vi "StressDist_plot.vi"(7 "StressDist_types":T8, 8 "Error In":errorcluster, 11 "main_FGV_data":T1={"pipe_properties"={"out_radius"=0.0, "in_radius"=0.0, "out_diameter"=0.0, "in_diameter"=0.0, "thickness"=0.0, "inertia"=0.0, "area"=0.0}, "DirPath"=path "L:/Documentos/00 SERVIÇOS/Tensão residual/Olapa 10-2017/Dados/Primeira Seção/Furos", "DirReport"=path "L:/Documentos/00 SERVIÇOS/Tensão residual/Olapa 10-2017/RelatóriosOlapa/Teste", "Points"=[], "ovalization_data"={"AngOval"=[0.0, 60.0, 120.0, 22.5, 45.0, 67.5, 90.0, 112.5, 135.0, 157.5, 180.0], "OvalDiam"=[324.25, 324.6, 324.55, 324.25, 324.55, 324.65, 324.6, 324.65, 324.55, 324.5, 324.4], "Plots"={"Ref"={"X"=[], "Y"=[]}, "Elipse"={"X"=[], "Y"=[]}, "Points"={"X"=[], "Y"=[]}}, "Ampliation"=100.0, "Results"={"MD"=0.0, "mD"=0.0, "Dmed"=0.0, "Oval"=0.0, "ang"=0.0, "X0"=0.0, "Y0"=0.0}}, "StressDist_data"={"Long"={"Plot"=[], "Fit"=[], "ColorMap"=[], "Data"=[], "peirce_data"={"Plot"=[], "Index removidos"=[]}}, "Circ"={"Plot"=[], "Fit"=[], "ColorMap"=[], "Data"=[], "peirce_data"={"Plot"=[], "Index removidos"=[]}}, "Shear"={"Plot"=[], "Fit"=[], "ColorMap"=[], "Data"=[], "peirce_data"={"Plot"=[], "Index removidos"=[]}}}}) -> (0 "Error Out":errorcluster, 3 "main_FGV_data-out":T1={"pipe_properties"={"out_radius"=0.0, "in_radius"=0.0, "out_diameter"=0.0, "in_diameter"=0.0, "thickness"=0.0, "inertia"=0.0, "area"=0.0}, "DirPath"=path "L:/Documentos/00 SERVIÇOS/Tensão residual/Olapa 10-2017/Dados/Primeira Seção/Furos", "DirReport"=path "L:/Documentos/00 SERVIÇOS/Tensão residual/Olapa 10-2017/RelatóriosOlapa/Teste", "Points"=[], "ovalization_data"={"AngOval"=[0.0, 60.0, 120.0, 22.5, 45.0, 67.5, 90.0, 112.5, 135.0, 157.5, 180.0], "OvalDiam"=[324.25, 324.6, 324.55, 324.25, 324.55, 324.65, 324.6, 324.65, 324.55, 324.5, 324.4], "Plots"={"Ref"={"X"=[], "Y"=[]}, "Elipse"={"X"=[], "Y"=[]}, "Points"={"X"=[], "Y"=[]}}, "Ampliation"=100.0, "Results"={"MD"=0.0, "mD"=0.0, "Dmed"=0.0, "Oval"=0.0, "ang"=0.0, "X0"=0.0, "Y0"=0.0}}, "StressDist_data"={"Long"={"Plot"=[], "Fit"=[], "ColorMap"=[], "Data"=[], "peirce_data"={"Plot"=[], "Index removidos"=[]}}, "Circ"={"Plot"=[], "Fit"=[], "ColorMap"=[], "Data"=[], "peirce_data"={"Plot"=[], "Index removidos"=[]}}, "Shear"={"Plot"=[], "Fit"=[], "ColorMap"=[], "Data"=[], "peirce_data"={"Plot"=[], "Index removidos"=[]}}}})   [LabVIEW 2016]
uses:
  StressDist_types.ctl
  MainFGV/main_FGV_data.ctl
  MainFGV/pipe_properties.ctl
  StressCalculations/point_data.ctl
  Ovalization/ovalization_data.ctl
  StressDist_data.ctl
  StressDist_single_data.ctl
  Peirce/peirce_data.ctl
  <vilib>/Analysis/1siggen.llb/Ramp Pattern by Samples.vi
  <vilib>/Analysis/NI_AALBase.lvlib
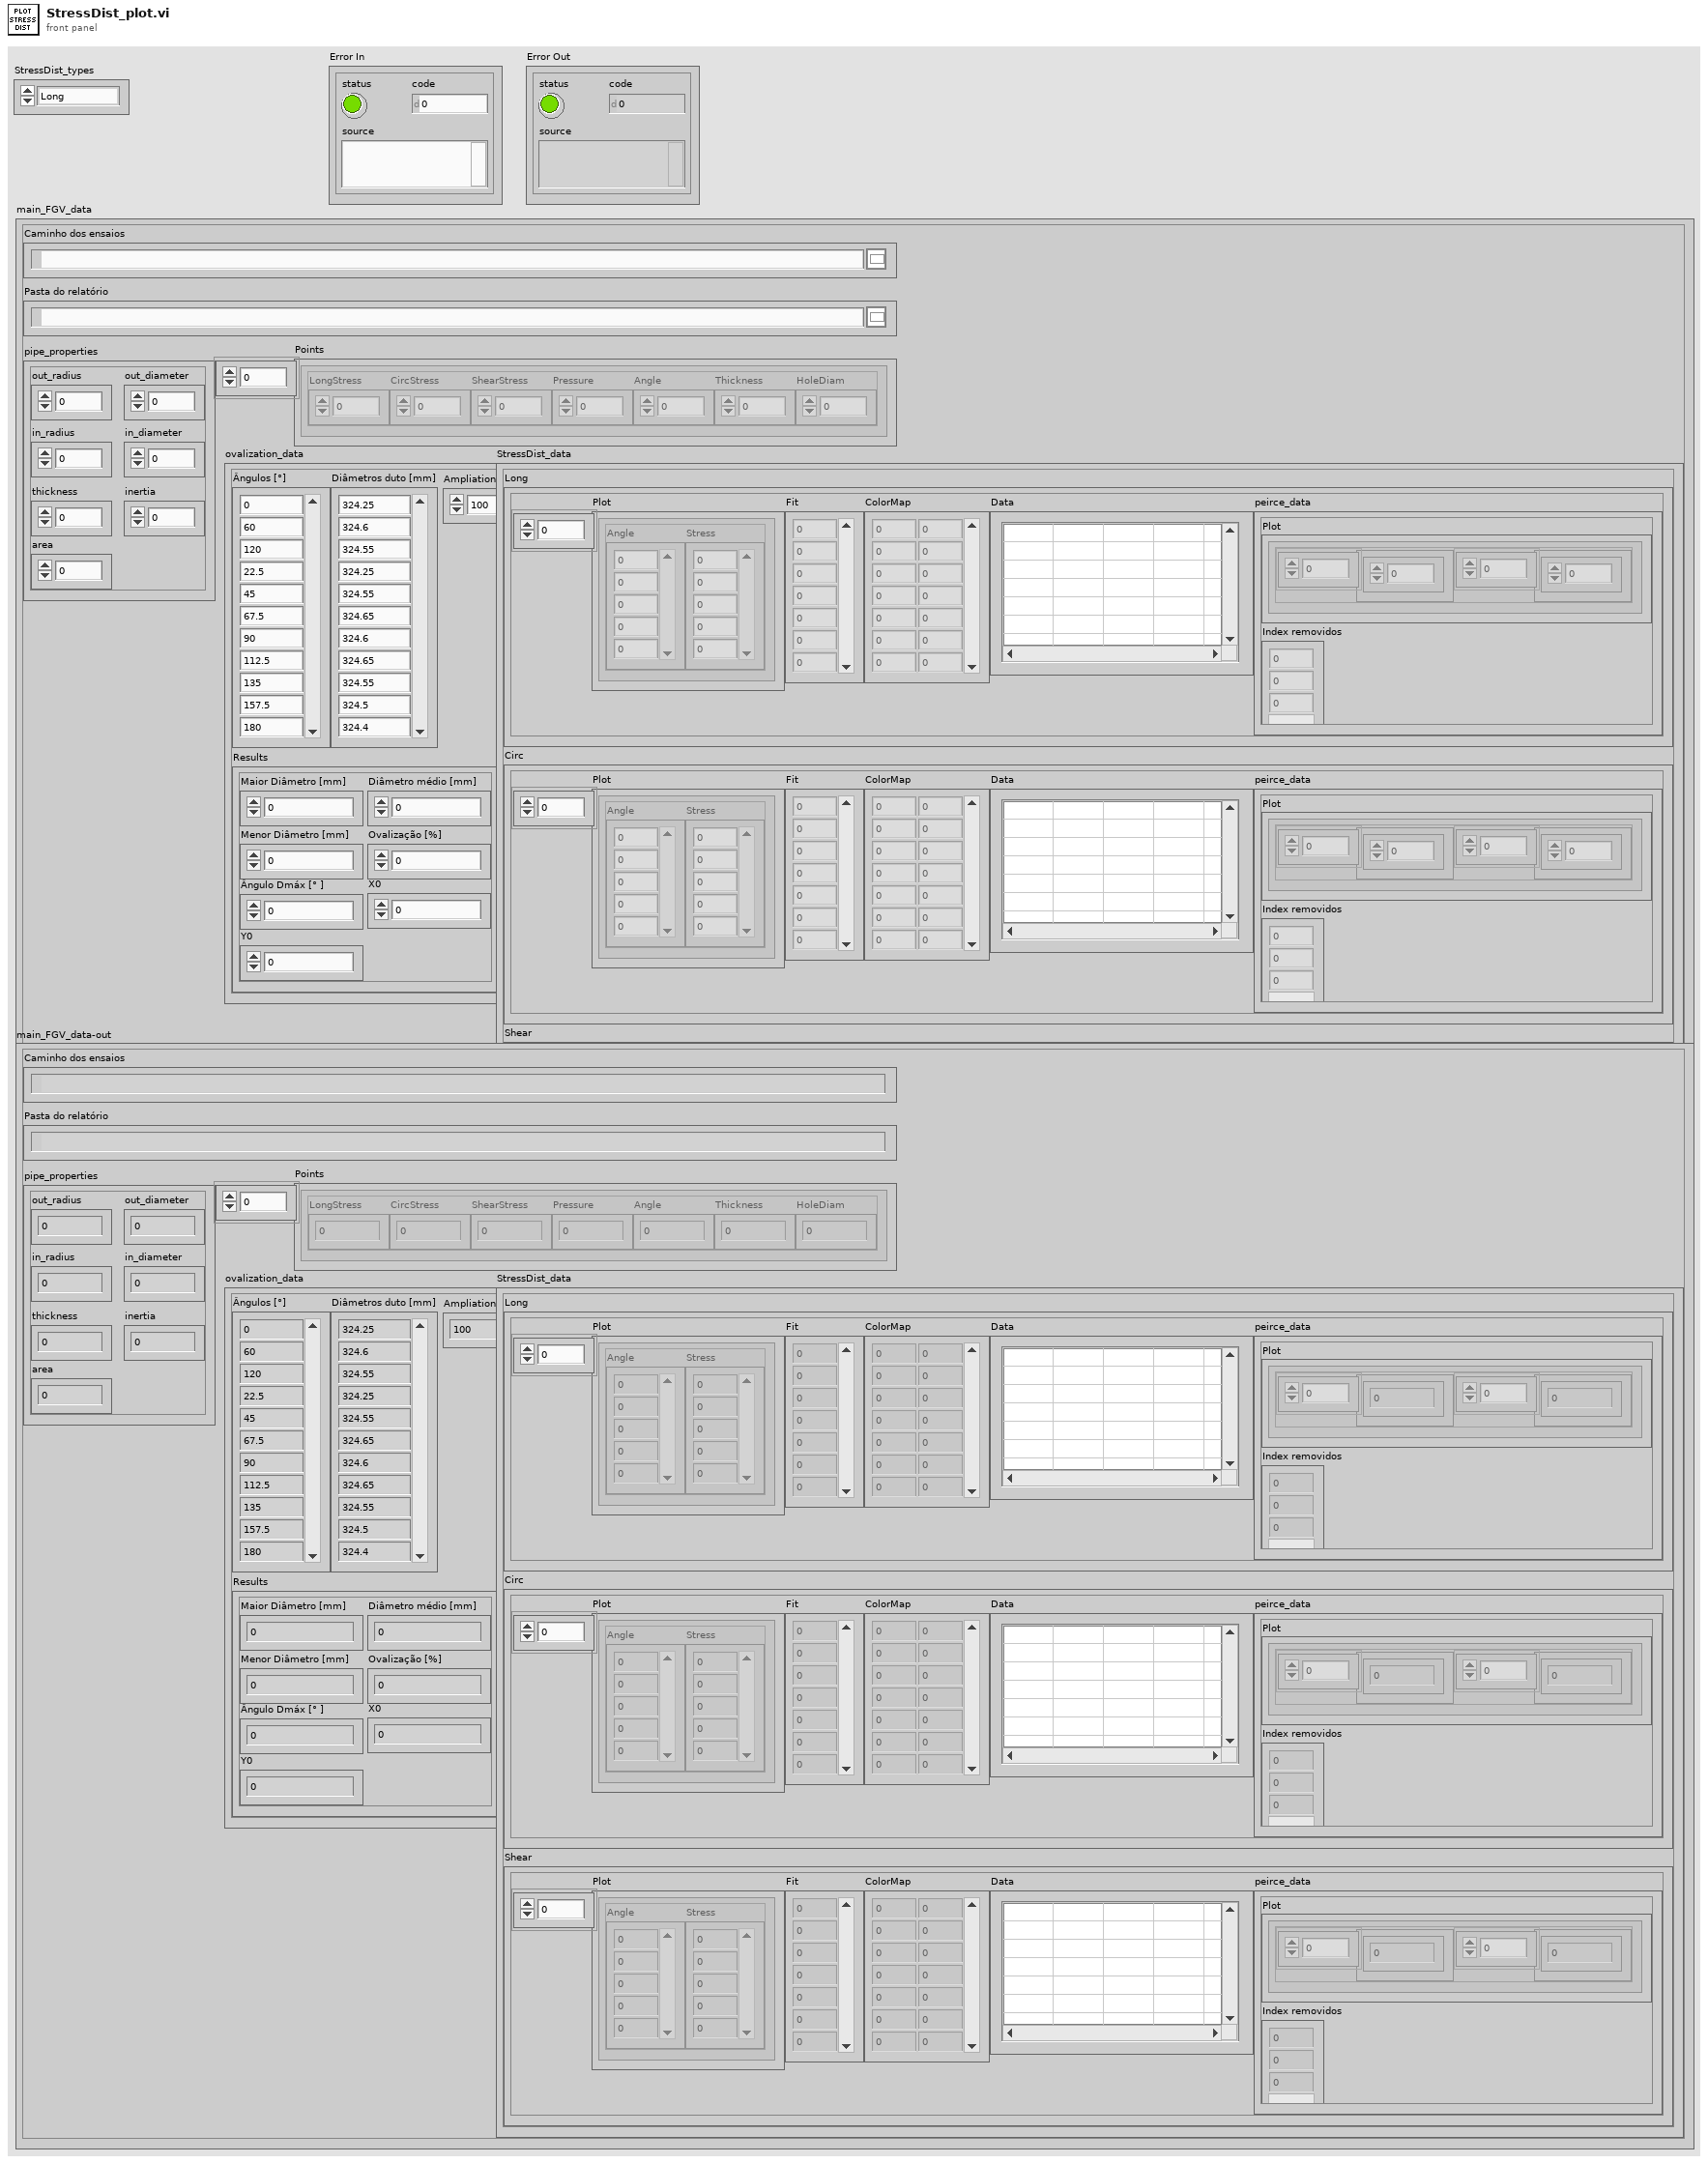
[diagram p1: front panel]
types:
  T1 = typedef "main_FGV_data.ctl" = cluster{"pipe_properties":T2, "DirPath":path, "DirReport":path, "Points":T3[], "ovalization_data":T4, "StressDist_data":T5}
  T2 = typedef "pipe_properties.ctl" = cluster{"out_radius":dbl, "in_radius":dbl, "out_diameter":dbl, "in_diameter":dbl, "thickness":dbl, "inertia":dbl, "area":dbl}
  T3 = typedef "point_data.ctl" = cluster{"LongStress":dbl, "CircStress":dbl, "ShearStress":dbl, "Pressure":dbl, "Angle":dbl, "Thickness":dbl, "HoleDiam":dbl}
  T4 = typedef "ovalization_data.ctl" = cluster{"AngOval":dbl[], "OvalDiam":dbl[], "Plots":cluster{"Ref":cluster{"X":dbl[], "Y":dbl[]}, "Elipse":cluster{"X":dbl[], "Y":dbl[]}, "Points":cluster{"X":dbl[], "Y":dbl[]}}, "Ampliation":dbl, "Results":cluster{"MD":dbl, "mD":dbl, "Dmed":dbl, "Oval":dbl, "ang":dbl, "X0":dbl, "Y0":dbl}}
  T5 = typedef "StressDist_data.ctl" = cluster{"Long":T6, "Circ":T6, "Shear":T6}
  T6 = typedef "StressDist_single_data.ctl" = cluster{"Plot":cluster{"Angle":dbl[], "Stress":dbl[]}[], "Fit":dbl[], "ColorMap":dbl[][], "Data":string[][], "peirce_data":T7}
  T7 = typedef "peirce_data.ctl" = cluster{"Plot":cluster{"Array":dbl[], "Array":dbl[]}[], "Index removidos":i32[]}
  T8 = typedef "StressDist_types.ctl" = enum16{"Long", "Circ", "Shear"}
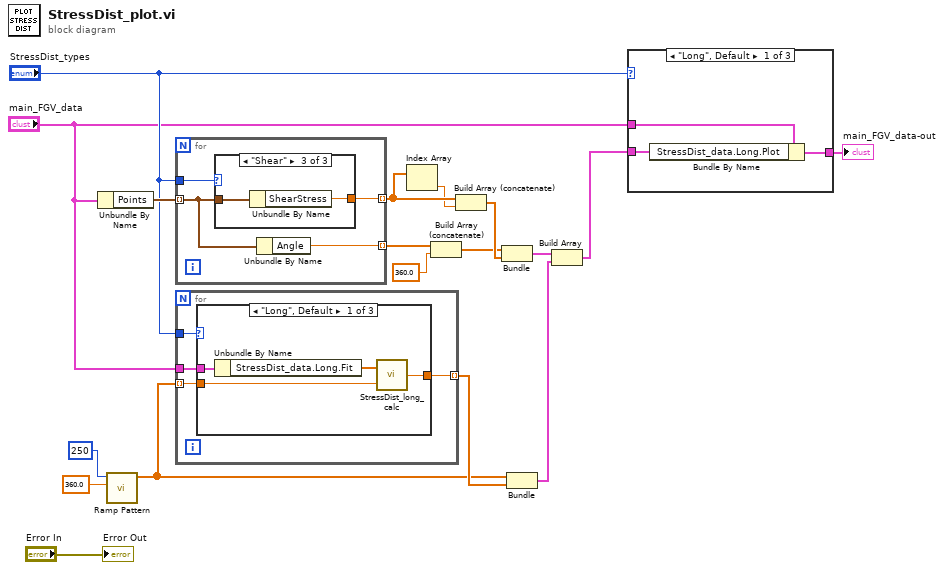
[diagram p0: block diagram]
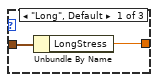
[diagram p2: hidden frame]
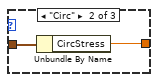
[diagram p3: hidden frame]
diagram:
  n1 = Unbundle By Name("main_FGV_data") -> ("Points"=w18:T3[])
  n2 = call-poly <vilib>:"Ramp Pattern.vi"("end"=360.0, "samples"=250) -> ("Ramp Pattern"=w15:dbl[])  [unwired: 8 in, 1 out]
  n3 = for {
    tunnel: "StressDist_types" -> [w22]
    tunnel: w18 -> [w21] mode=indexing
    tunnel: [w20] -> w5 mode=indexing
    tunnel: [w19] -> w7 mode=indexing
    n4 = case shown="\"Shear\"" w22 {
      tunnel: w21 -> [w24 w26 w28]
      tunnel: [w23 w25 w27] -> w20
      frame "Long", Default {
        n5 = Unbundle By Name(w24) -> ("LongStress"=w23:dbl)
      }
      frame "Circ" {
        n6 = Unbundle By Name(w26) -> ("CircStress"=w25:dbl)
      }
      frame "Shear" {
        n7 = Unbundle By Name(w28) -> ("ShearStress"=w27:dbl)
      }
    }
    n8 = Unbundle By Name(w21) -> ("Angle"=w19:dbl)
  }
  n9 = for {
    tunnel: "StressDist_types" -> [w32]
    tunnel: w15 -> [w31] mode=indexing
    tunnel: [w30] -> w16 mode=indexing
    tunnel: "main_FGV_data" -> [w29]
    n10 = case shown="\"Long\", Default" w32 {
      tunnel: w31 -> [w36 _ _]
      tunnel: [w35 _ _] -> w30
      tunnel: w29 -> [w34 _ _]
      frame "Long", Default {
        n11 = Unbundle By Name(w34) -> ("StressDist_data.Long.Fit"=w33:dbl[])
        n12 = call "StressDist_long_calc.vi"("Angle"=w36, "Parameters"=w33) -> ("Stress"=w35:dbl)
      }
      frame "Circ" {
      }
      frame "Shear" {
      }
    }
  }
  n13 = Index Array(array=w5) -> (element=w4:dbl)  [unwired: 1 in]
  n14 = Build Array (concatenate)(w7, 360.0 ("end")) -> (w2:dbl[])
  n15 = Build Array (concatenate)(w5, w4) -> (w3:dbl[])
  n16 = Bundle(w2, w3) -> (w14:cluster{dbl[], dbl[]})  [unwired: 1 in]
  n17 = Bundle("Ramp Pattern"=w15, w16) -> (w13:cluster{"Ramp Pattern":dbl[], dbl[]})  [unwired: 1 in]
  n18 = Build Array(w14, w13) -> (w10:cluster{"Ramp Pattern":dbl[], dbl[]}[])
  n19 = case shown="\"Long\", Default" "StressDist_types" {
    tunnel: "main_FGV_data" -> [w39 _ _]
    tunnel: w10 -> [w38 _ _]
    tunnel: [w37 _ _] -> w9
    frame "Long", Default {
      n20 = Bundle By Name(cluster=w39, "StressDist_data.Long.Plot"=w38) -> (w37:T1)
    }
    frame "Circ" {
    }
    frame "Shear" {
    }
  }
  "main_FGV_data-out" <- w9
  "Error Out" <- "Error In"
